vi "Read Write Registers.vi"(5 "Read Count":u16, 6 "timeout ms (1000)":i32=1000, 7 "Read Start Address":u16, 8 "error in (no error)":errorcluster, 9 "Write Values":u16[](array[numeric]), 10 "Write Start Address":u16, 11 "TCP Network Connection in":refnum<k5>) -> (0 "error out":errorcluster, 1 "Read Values":u16[](array[numeric]), 3 "TCP Network Connection out":refnum<k5>)   [LabVIEW 2023, in "Modbus TCP Micro.lvlib"]
uses:
  Modbus TCP Micro.lvlib
  Modbus Functions.ctl
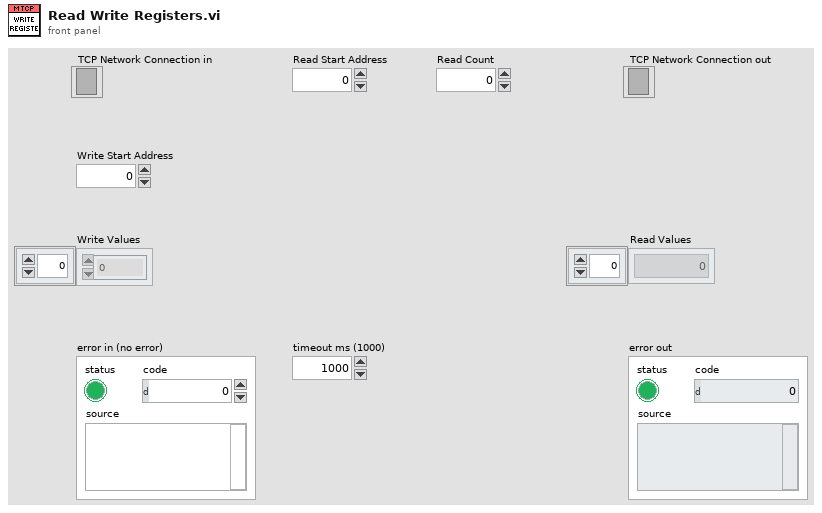
[diagram p1: front panel]
types:
  T1 = typedef "Modbus TCP Micro.lvlib/Modbus Functions.ctl" = u8
  T2 = cluster{"Read Count":u16, "Write Start Address":u16, u16, u8}
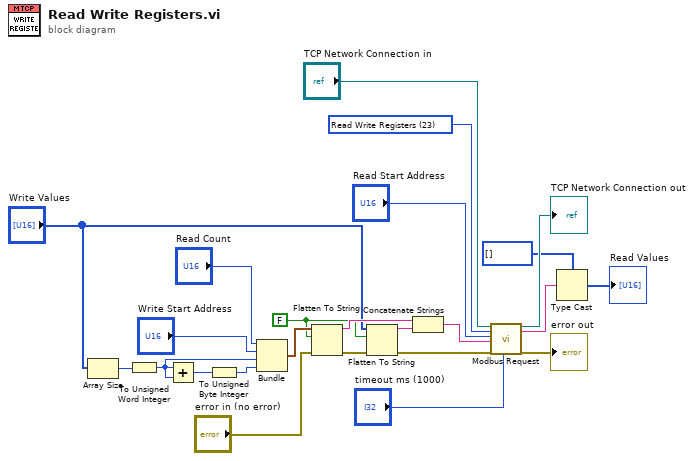
[diagram p0: block diagram]
diagram:
  w8 = T1 23 items=["None"=0, "Read Coil Status"=1, "Read Input Status"=2, "Read Holding Registers"=3, "Read Input Registers"=4, "Force Single Coil"=5, "Preset Single Register"=6, "Force Multiple Coils"=15, "Preset Multiple Registers"=16, "Mask Write Register"=22, "Read Write Registers"=23] ("Function Codes")
  w11 = FALSE ("prepend array or string size? (T)")
  n1 = Array Size(array="Write Values") -> (size(s)=w19:i32)
  n2 = To Unsigned Word Integer(number=w19) -> (unsigned 16bit integer=w18:u16)
  n3 = Add(x=w18, y=w18) -> (x+y=w17:u16)
  n4 = To Unsigned Byte Integer(number=w17) -> (unsigned 8bit integer=w16:u8)
  n5 = Bundle("Read Count"="Read Count", "Write Start Address"="Write Start Address", w18, w16) -> (w15:T2)  [unwired: 1 in]
  n6 = Flatten To String(anything=w15, prepend array or string size? (T)=w11, error in (no error)="error in (no error)") -> (data string=w20:string, error out=w10:errorcluster)  [unwired: 1 in, 1 out]
  n7 = Flatten To String(anything="Write Values", prepend array or string size? (T)=w11, error in (no error)=w10) -> (data string=w12:string, error out=w9:errorcluster)  [unwired: 1 in, 1 out]
  n8 = Concatenate Strings(w20, w12) -> (w13:string)
  n9 = call "Modbus Request.vi"("TCP Network Connection in"="TCP Network Connection in", "Function Codes"=w8, "Start Address"="Read Start Address", "Payload"=w13, "error in (no error)"=w9, "timeout ms (1000)"="timeout ms (1000)") -> ("TCP Network Connection out"=→"TCP Network Connection out":refnum<k5>, "Payload"=w6:string, "error out"=→"error out":errorcluster)  [unwired: 8 in, 3 out]
  n10 = Type Cast(type=u16[] [], x=w6) -> (*(type *) &x=→"Read Values":u16[])
